vi "Close.vi"(8 "error in":errorcluster, 11 "MyEventGrid in":refnum<class "MyEventGrid.lvclass">) -> (0 "error out":errorcluster, 3 "MyEventGrid out":refnum<class "MyEventGrid.lvclass">)   [LabVIEW 2023, in "MyEventGrid.lvclass"]
uses:
  MyEventGrid.lvclass
  MyEventGrid.lvclass/MyEventGrid.ctl
  source/Grid/SourceGrid.lvclass
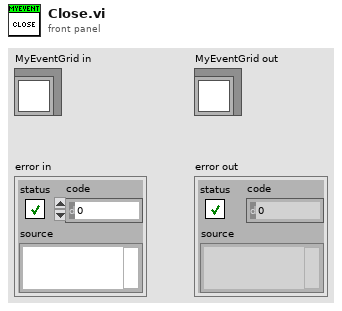
[diagram p1: front panel]
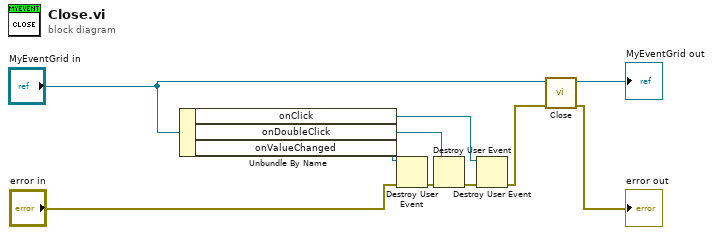
[diagram p0: block diagram]
diagram:
  n1 = Unbundle By Name("MyEventGrid in") -> ("onClick"=w8:refnum<user-event>, "onDoubleClick"=w7:refnum<user-event>, "onValueChanged"=w5:refnum<user-event>)
  n2 = Destroy User Event(user event=w5, error in="error in") -> (error out=w6:errorcluster)
  n3 = Destroy User Event(user event=w7, error in=w6) -> (error out=w9:errorcluster)
  n4 = Destroy User Event(user event=w8, error in=w9) -> (error out=w1:errorcluster)
  n5 = call-parent "Close.vi"("error in"=w1, "Sourcegrid in"="MyEventGrid in") -> ("error out"=→"error out":errorcluster, "Sourcegrid out"=→"MyEventGrid out":refnum<class "MyEventGrid.lvclass">)  [unwired: 8 in]
